vi "LoadCustomGlyphs.vi"(7 "tree ref":refnum<vi>, 8 "error in":errorcluster, 11 "glyph directory":path) -> (0 "error out":errorcluster)   [LabVIEW 2013, in "NISE_CEF_TreeControl.lvlib"]
doc: "Adds the glyphs in the folder glyph to the tree control, so nodes can use it. \nThe default behaivior is that it will search for all the glyphs on the Glyph folder. It wont do search for directories inside of it. \nAnd file names are NOT Case sensitive."
uses:
  NISE_CEF_TreeControl.lvlib
  Controls/GlyphIndexPair.ctl
  Controls/GlyphIndexPairActions.ctl
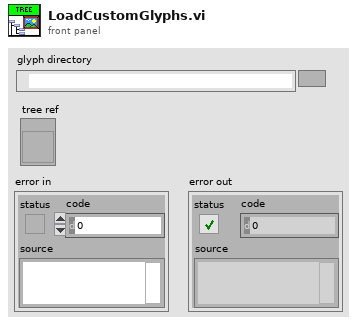
[diagram p1: front panel]
types:
  T1 = typedef "NISE_CEF_TreeControl.lvlib/GlyphIndexPairActions.ctl" = enum16{"Get", "Initialize"}
  T2 = typedef "NISE_CEF_TreeControl.lvlib/GlyphIndexPair.ctl" = cluster{"name":string, "index":i32}
  T3 = typedef "imagedata.ctl" = cluster{"image type":i32, "image depth":i32, "image":u8[], "mask":u8[], "colors":u32[], "Rectangle":cluster{"left":i16, "top":i16, "right":i16, "bottom":i16}}
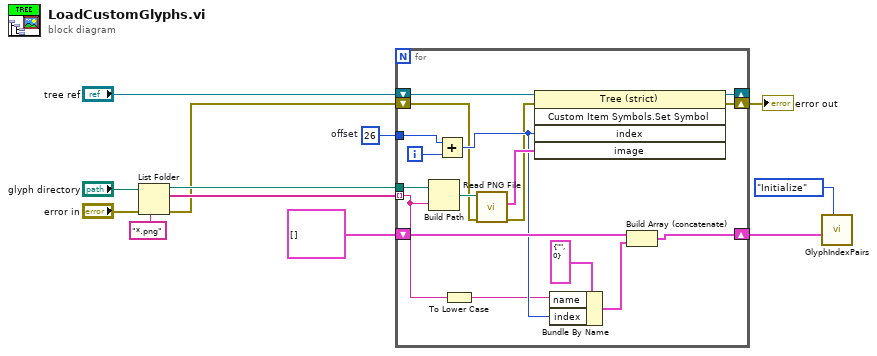
[diagram p0: block diagram]
diagram:
  w6 = 26  # offset
  n1 = List Folder(path="glyph directory", pattern="*.png", error in="error in") -> (path out=w9:path, filenames=w8:string[], error out=w5:errorcluster)  [unwired: 1 in, 1 out]
  n2 = for {
    tunnel: w9 -> [w29]
    tunnel: w8 -> [w14] mode=indexing
    shift-right: [w27] -> _
    shift-left: "tree ref" -> [w28]
    tunnel: w6 -> [w23]
    shift-right: [w18] -> w4
    shift-left: w5 -> [w16]
    shift-right: [w19] -> w2
    shift-left: T2[] [] ("array") -> [w22]
    i -> [w24]
    n3 = Build Path(base path=w29, name or relative path=w14) -> (appended path=w26:path)
    n4 = Add(x=w23, y=w24) -> (x+y=w20:i32)
    n5 = To Lower Case(string=w14) -> (all lower case string=w13:string)
    n6 = call <vilib>:"Read PNG File.vi"("error in (no error)"=w16, "path to PNG file"=w26) -> ("error out"=w15:errorcluster, "image data"=w25:T3)  [unwired: 7 in, 1 out]
    n7 = invoke class="Tree (strict)" method="Custom Item Symbols.Set Symbol"(reference=w28, error in=w15, "index"=w20, "image"=w25) -> (reference out=w27:refnum<vi>, error out=w18:errorcluster)  [unwired: 1 in, 3 out]
    n8 = Bundle By Name(cluster=T2 {"name"="", "index"=0} ("glyphIndexPair"), "name"=w13, "index"=w20) -> (w21:T2)
    n9 = Build Array (concatenate)(w22, w21) -> (w19:T2[])
  }
  "error out" <- w4
  n10 = call "GlyphIndexPairs.vi"("action"=GlyphIndexPairActions."Initialize" ("Enum"), "array"=w2) -> ()  [unwired: 8 in, 2 out]
